vi "Remove-action.vi"(8 "error in (no error)":errorcluster, 9 "Position in":i32, 11 "Sequence in":refnum<class "Action-sequence.lvclass">) -> (0 "error out":errorcluster, 1 "Position":i32, 2 "Removed action":refnum<class "Action.lvclass">, 3 "Sequence out":refnum<class "Action-sequence.lvclass">)   [LabVIEW 2013, in "PowderDeposition.lvlib" / "Action-sequence.lvclass"]
uses:
  Action-sequence.lvclass
  Action/Action.lvclass
  Action-sequence.lvclass/Action-sequence.ctl
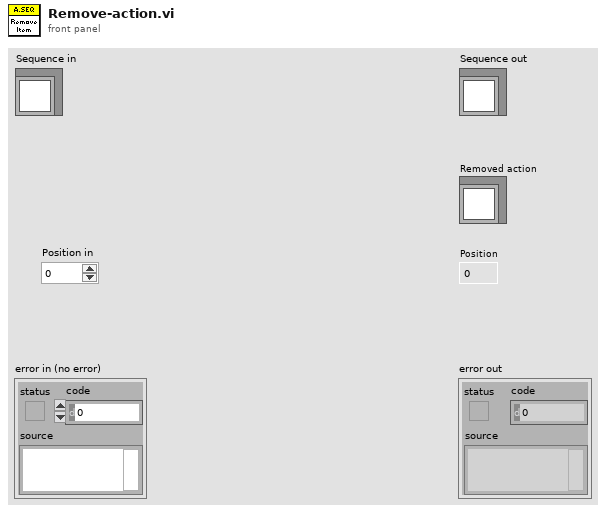
[diagram p1: front panel]
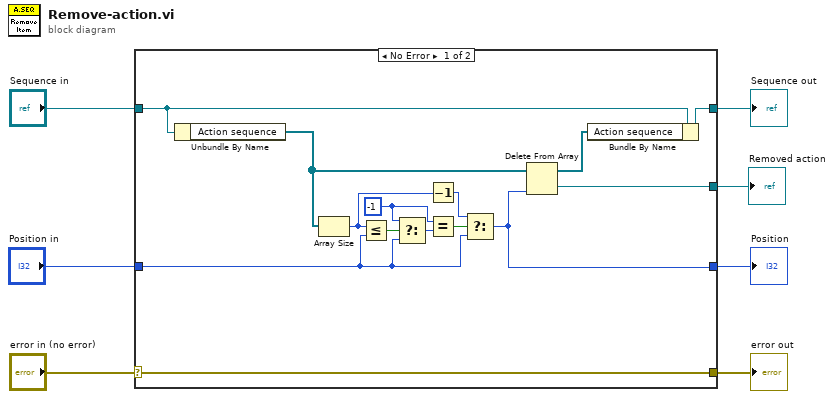
[diagram p0: block diagram]
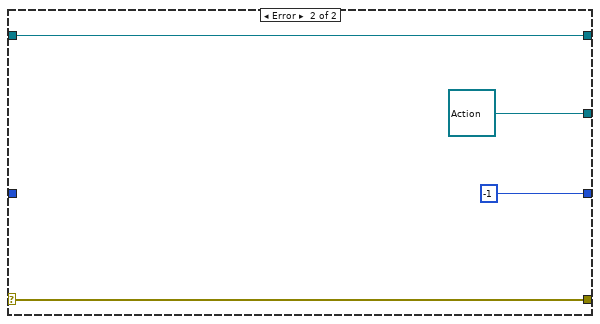
[diagram p2: hidden frame]
diagram:
  n1 = case shown="No Error" "error in (no error)" {
    selector: "error in (no error)" -> [w11 w25]
    tunnel: [w11 w25] -> w6
    tunnel: [w21 w24] -> w4
    tunnel: "Sequence in" -> [w8 w24]
    tunnel: "Position in" -> [w14 _]
    tunnel: [w12 -1 ("Position")] -> w2
    tunnel: [w9 refnum<class "Action.lvclass"> refnum ("Action.lvclass")] -> w1
    frame No Error {
      w18 = -1 ("t")
      n2 = Unbundle By Name(w8) -> ("Action sequence"=w13:refnum<class "Action.lvclass">[])
      n3 = Array Size(array=w13) -> (size(s)=w16:i32)
      n4 = Less Or Equal?(x=w16, y=w14) -> (x <= y?=w20:bool)
      n5 = Select(t=w18, s=w20, f=w14) -> (s? t:f=w19:i32)
      n6 = Decrement(x=w16) -> (x-1=w15:i32)
      n7 = Equal?(x=w18, y=w19) -> (x = y?=w17:bool)
      n8 = Select(t=w15, s=w17, f=w14) -> (s? t:f=w12:i32)
      n9 = Delete From Array(array=w13, index=w12) -> (deleted portion=w9:refnum<class "Action.lvclass">, array with subset deleted=w10:refnum<class "Action.lvclass">[])  [unwired: 1 in]
      n10 = Bundle By Name(cluster=w8, "Action sequence"=w10) -> (w21:refnum<class "Action-sequence.lvclass">)
    }
    frame Error {
    }
  }
  "error out" <- w6
  "Sequence out" <- w4
  "Removed action" <- w1
  "Position" <- w2
